vi "Misc-Query Instrument State.vi"(0 "VISA resource name":refnum<visa-resource-name>, 11 "error in (no error)":errorcluster) -> (4 "VISA resource name out":refnum<visa-resource-name>, 10 "state (unknown:0)":u16(ring) items=["unknown", "idle", "standby", "measurement", "stress force"], 15 "error out":errorcluster)   [LabVIEW 2016, in "Agilent 415X Series.lvlib"]
doc: "This VI queries the instrument for its present state which can be\n 1 - Idle\n 2 - Standby\n 3 - Measurement\n 4 - Stress Force\n\nIn case of a Read Error, 0 (Unknown) will be returned."
uses:
  Agilent 415X Series.lvlib
panel:
  in  "pattern":string[](array[string])=["XXX", "I", "S", "M", "S"]
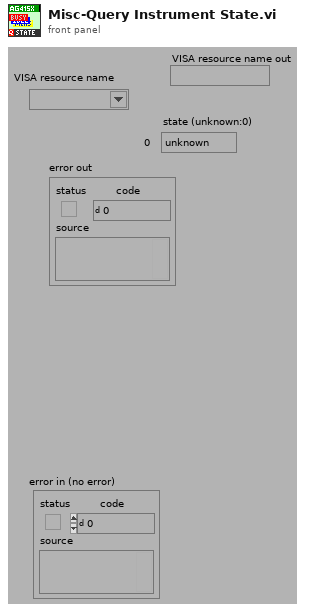
[diagram p1: front panel]
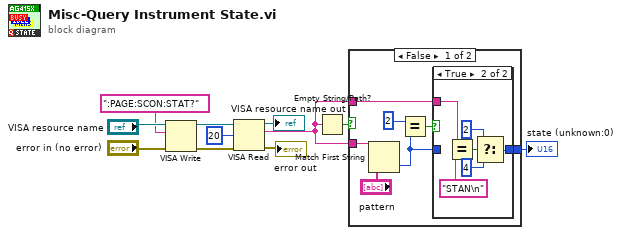
[diagram p0: block diagram]
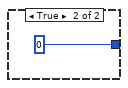
[diagram p3: hidden frame]
diagram:
  n1 = VISA Write(VISA resource name="VISA resource name", write buffer=":PAGE:SCON:STAT?", error in (no error)="error in (no error)") -> (VISA resource name out=w7:refnum<visa-resource-name>, error out=w8:errorcluster)  [unwired: 1 out]
  n2 = VISA Read(VISA resource name=w7, byte count=u32 20, error in (no error)=w8) -> (VISA resource name out=→"VISA resource name out":refnum<visa-resource-name>, read buffer=w2:string, error out=→"error out":errorcluster)  [unwired: 1 out]
  n3 = Empty String/Path?(string/path=w2) -> (empty?=w4:bool)
  n4 = case shown="False" w4 {
    tunnel: [w13 0] -> w3
    tunnel: w2 -> [w17 _]
    tunnel: w2 -> [w12 _]
    frame False {
      n5 = Match First String(2:"pattern", 3:w17) -> (0:w14:i32)  [unwired: 1 out]
      n6 = Equal?(x=2, y=w14) -> (x = y?=w15:bool)
      n7 = case shown="True" w15 {
        tunnel: w14 -> [w19 _]
        tunnel: [w19 w22] -> w13
        tunnel: w12 -> [_ w20]
        frame False {
        }
        frame True {
          n8 = Equal?(x=w20, y="STAN\n") -> (x = y?=w21:bool)
          n9 = Select(t=2, s=w21, f=4) -> (s? t:f=w22:i32)
        }
      }
    }
    frame True {
    }
  }
  "state (unknown:0)" <- w3
